vi "process.vi"(8 "error in (no error)":errorcluster, 11 "ConnectionHandler in":refnum<class "ConnectionHandler.lvclass">) -> (0 "error out":errorcluster, 3 "ConnectionHandler":refnum<class "ConnectionHandler.lvclass">)   [LabVIEW 2013, in "MQTT Server.lvlib" / "ConnectionHandler.lvclass"]
uses:
  ConnectionHandler.lvclass
  <vilib>/LabVIEW Open Source Project/MQTT Connection/MQTT_Base/Session/Session.lvclass
  ConnectionHandler.lvclass/ConnectionHandler.ctl
  Session.Server/Session.Server.lvclass
  <vilib>/LabVIEW Open Source Project/MQTT Connection/MQTT_Base/Session/Session.lvclass/Session.ctl
  <vilib>/Utility/error.llb/Clear Errors.vi
  <vilib>/LabVIEW Open Source Project/MQTT Connection/MQTT_Connection/Connection/Connection.lvclass
panel:
  out "Stored Connections":i32
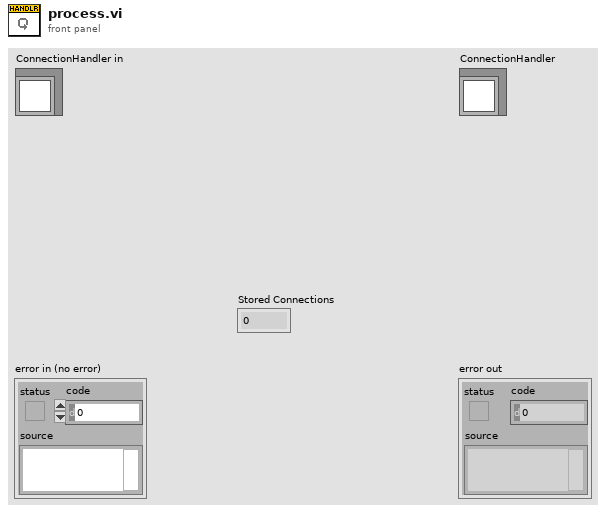
[diagram p1: front panel]
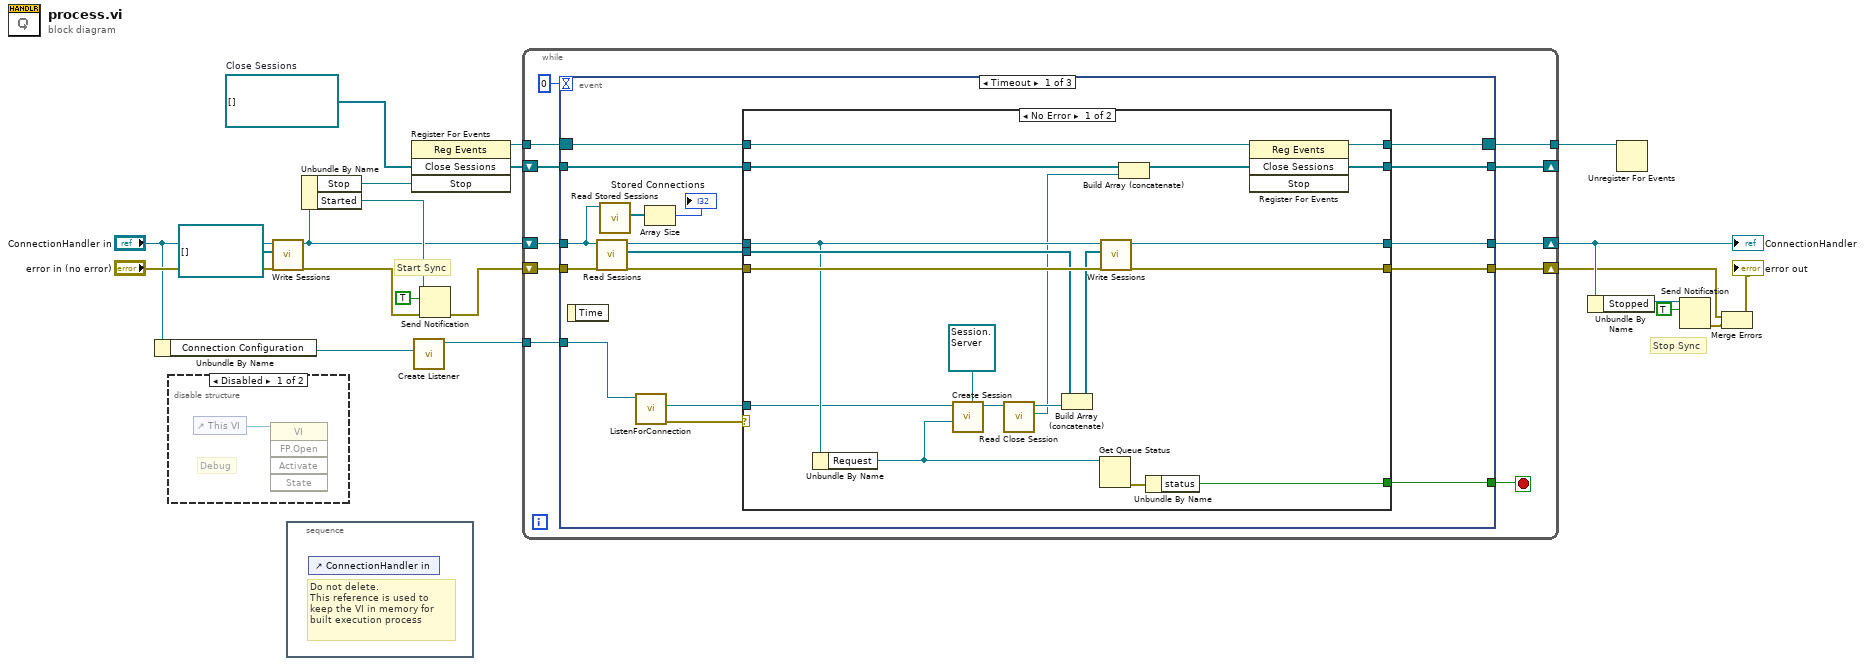
[diagram p0: block diagram]
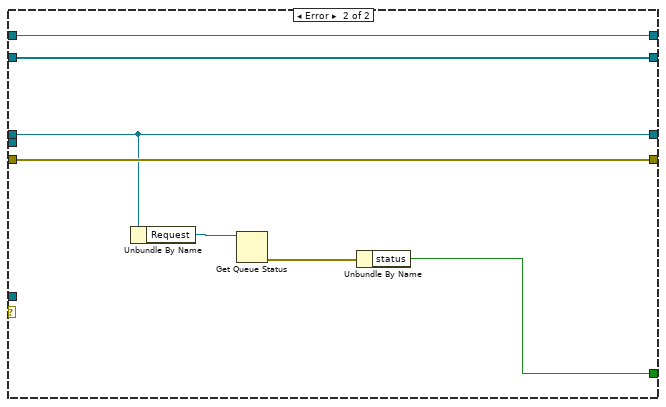
[diagram p3: hidden frame]
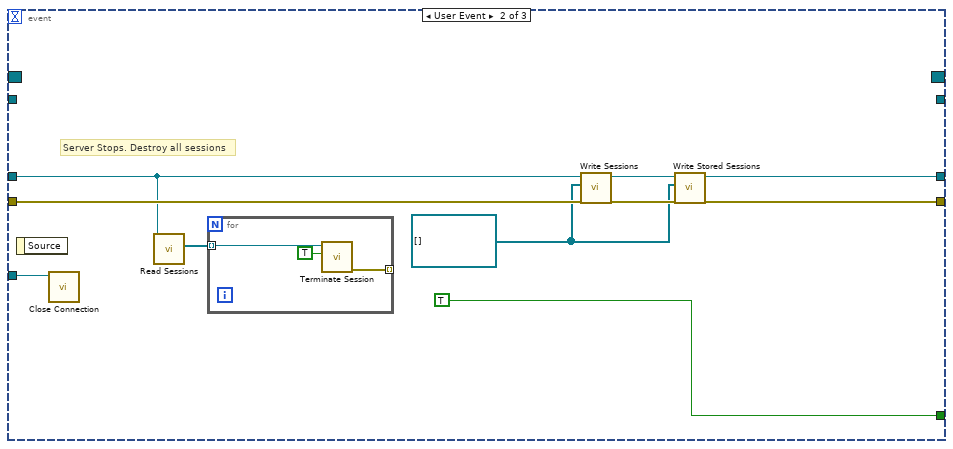
[diagram p4: hidden frame]
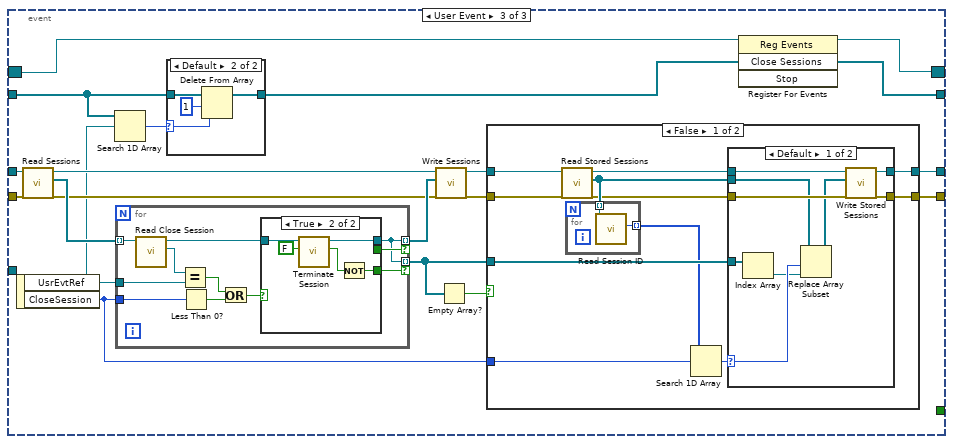
[diagram p5: hidden frame]
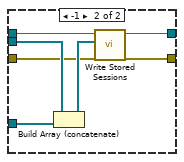
[diagram p7: hidden frame]
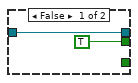
[diagram p9: hidden frame]
diagram:
  w4 = refnum<user-event>[] []  # Close Sessions
  # "Stop Sync"
  # "Start Sync"
  n1 = Unbundle By Name("ConnectionHandler in") -> ("Connection Configuration"=w6:refnum<class "Connection.lvclass">)
  n2 = disable-structure shown="Disabled" {
    frame Disabled {
      # "Debug"
      n3 = control-ref of="This VI"() -> (w20:refnum<vi>)
      n4 = invoke class="VI" method="FP.Open"(reference=w20) -> ()  [unwired: 4 in, 5 out]
    }
    frame Enabled {
    }
  }
  n5 = call "Write Sessions.vi"("Sessions"=refnum<class "Session.lvclass">[] [], "ConnectionHandler in"="ConnectionHandler in") -> ("ConnectionHandler"=w2:refnum<class "ConnectionHandler.lvclass">)  [unwired: 9 in]
  n6 = stacked-sequence {
    frame #0 {
      # "Do not delete.\nThis reference is used to keep the VI in memory for built execution process"
      n7 = control-ref of="ConnectionHandler in"() -> ()  [unwired: 1 out]
    }
  }
  n8 = Unbundle By Name(w2) -> ("Stop"=w19:refnum<user-event>, "Started"=w14:refnum<notifier>)
  n9 = register-events(w4, w19) -> (reference out=w17:refnum<event-registration>)  [unwired: 2 in, 1 out]
  n10 = call <vilib>:"Create Listener.vi"("Connection Configuration"=w6) -> ("Listener"=w5:refnum<class "Connection.lvclass">)  [unwired: 9 in, 1 out]
  n11 = Send Notification(notification=TRUE, notifier=w14, error in (no error)="error in (no error)") -> (error out=w15:errorcluster)  [unwired: 1 out]
  n12 = while {
    shift-right: [w28] -> w13
    shift-left: w2 -> [w27]
    shift-right: [w30] -> w8
    shift-left: w15 -> [w29]
    tunnel: w17 -> [w26]
    tunnel: [w25] -> w18
    tunnel: w5 -> [w23]
    shift-right: [w22] -> _
    shift-left: w4 -> [w21]
    stop <- w24 stop-if-true
    n13 = event shown="[0] Timeout" {
      selector: w26 -> [w35 _ w86]
      dyn-events: [w34 _ w87] -> w25
      timeout: 0 -> [_ _ _]
      tunnel: [w45 w79 w91] -> w30
      tunnel: w29 -> [w47 w79 w90]
      tunnel: [w46 w74 w97] -> w28
      tunnel: w27 -> [w41 w76 w95]
      tunnel: [w44 TRUE _] -> w24
      tunnel: w23 -> [w37 w72 _]
      tunnel: [w33 _ w83] -> w22
      tunnel: w21 -> [w32 _ w85]
      event Timeout {
        n14 = event-data() -> ()  [unwired: 1 in, 1 out]
        n15 = call "Read Sessions.vi"("ConnectionHandler in"=w41) -> ("Sessions"=w42:refnum<class "Session.lvclass">[], "ConnectionHandler"=w43:refnum<class "ConnectionHandler.lvclass">)  [unwired: 9 in]
        n16 = call "Read Stored Sessions.vi"("ConnectionHandler in"=w41) -> ("Stored Sessions"=w40:refnum<class "Session.lvclass">[])  [unwired: 9 in, 1 out]
        n17 = call <vilib>:"ListenForConnection.vi"("Listener"=w37) -> ("error out"=w38:errorcluster, "Connection"=w39:refnum<class "Connection.lvclass">)  [unwired: 7 in, 2 out]
        n18 = Array Size(array=w40) -> (size(s)=→"Stored Connections":i32)
        n19 = case shown="No Error" w38 {
          tunnel: w43 -> [w59 w70]
          tunnel: w47 -> [w64 w71]
          tunnel: [w63 w70] -> w46
          tunnel: [w64 w71] -> w45
          tunnel: [w61 w67] -> w44
          tunnel: w42 -> [w60 _]
          tunnel: w39 -> [w57 _]
          tunnel: w35 -> [w55 w66]
          tunnel: [w54 w66] -> w34
          tunnel: [w48 w65] -> w33
          tunnel: w32 -> [w49 w65]
          frame No Error {
            n20 = Unbundle By Name(w59) -> ("Request"=w56:refnum<queue>)
            n21 = call <vilib>:"Create Session.vi"("Session in"=refnum<class "Session.Server.lvclass"> refnum ("MQTT Server.lvlib:Session.Server.lvclass"), "Request"=w56, "Connection"=w57) -> ("Session"=w52:refnum<class "Session.Server.lvclass">)  [unwired: 7 in, 1 out]
            n22 = call <vilib>:"Read Close Session.vi"("Session in"=w52) -> ("Close Session"=w50:refnum<user-event>, "Session out"=w51:refnum<class "Session.Server.lvclass">)  [unwired: 8 in, 1 out]
            n23 = Build Array (concatenate)(w60, w51) -> (w53:refnum<class "Session.lvclass">[])
            n24 = Get Queue Status(queue=w56) -> (error out=w62:errorcluster)  [unwired: 2 in, 7 out]
            n25 = call "Write Sessions.vi"("Sessions"=w53, "ConnectionHandler in"=w59) -> ("ConnectionHandler"=w63:refnum<class "ConnectionHandler.lvclass">)  [unwired: 9 in]
            n26 = Build Array (concatenate)(w49, w50) -> (w48:refnum<user-event>[])
            n27 = Unbundle By Name(w62) -> ("status"=w61:bool)
            n28 = register-events(reference=w55, w48) -> (reference out=w54:refnum<event-registration>)  [unwired: 2 in, 1 out]
          }
          frame Error {
            n29 = Unbundle By Name(w70) -> ("Request"=w69:refnum<queue>)
            n30 = Get Queue Status(queue=w69) -> (error out=w68:errorcluster)  [unwired: 2 in, 7 out]
            n31 = Unbundle By Name(w68) -> ("status"=w67:bool)
          }
        }
      }
      event User Event {
        w73 = refnum<class "Session.lvclass">[] [] ("Sessions")
        # "Server Stops. Destroy all sessions"
        n32 = event-data() -> ()  [unwired: 1 in, 1 out]
        n33 = call <vilib>:"Close Connection.vi"("Connection in"=w72) -> ()  [unwired: 9 in, 2 out]
        n34 = call "Read Sessions.vi"("ConnectionHandler in"=w76) -> ("Sessions"=w77:refnum<class "Session.lvclass">[])  [unwired: 9 in, 1 out]
        n35 = for {
          tunnel: w77 -> [w82] mode=indexing
          tunnel: [w81] -> _ mode=indexing
          n36 = call <vilib>:"Terminate Session.vi"("Destroy (T)"=TRUE, "Session in"=w82) -> ("error out"=w81:errorcluster)  [unwired: 7 in, 2 out]
        }
        n37 = call "Write Sessions.vi"("Sessions"=w73, "ConnectionHandler in"=w76) -> ("ConnectionHandler"=w75:refnum<class "ConnectionHandler.lvclass">)  [unwired: 9 in]
        n38 = call "Write Stored Sessions.vi"("Stored Sessions"=w73, "ConnectionHandler in"=w75) -> ("ConnectionHandler"=w74:refnum<class "ConnectionHandler.lvclass">)  [unwired: 9 in]
      }
      event User Event {
        n39 = event-data() -> ("UsrEvtRef"=w88:refnum<user-event>, "CloseSession"=w89:i32)  [unwired: 1 in]
        n40 = call "Read Sessions.vi"("ConnectionHandler in"=w95) -> ("Sessions"=w99:refnum<class "Session.lvclass">[], "ConnectionHandler"=w94:refnum<class "ConnectionHandler.lvclass">)  [unwired: 9 in]
        n41 = Search 1D Array(1D array=w85, element=w88) -> (index of element=w84:i32)  [unwired: 1 in]
        n42 = for {
          tunnel: w99 -> [w133] mode=indexing
          tunnel: [w139] -> w98 mode=indexing if=w143
          tunnel: w89 -> [w141]
          tunnel: [w139] -> w93 mode=indexing if=w138
          tunnel: w88 -> [w136]
          n43 = call <vilib>:"Read Close Session.vi"("Session in"=w133) -> ("Close Session"=w134:refnum<user-event>, "Session out"=w137:refnum<class "Session.lvclass">)  [unwired: 8 in, 1 out]
          n44 = Equal?(x=w134, y=w136) -> (x = y?=w135:bool)
          n45 = Less Than 0?(x=w141) -> (x < 0?=w142:bool)
          n46 = Or(x=w135, y=w142) -> (x .or. y?=w140:bool)
          n47 = case shown="True" w140 {
            tunnel: w137 -> [w145 w150]
            tunnel: [w145 w149] -> w139
            tunnel: [TRUE _] -> w143
            tunnel: [_ w146] -> w138
            frame False {
            }
            frame True {
              n48 = call <vilib>:"Terminate Session.vi"("Destroy (T)"=FALSE, "Session in"=w150) -> ("Destroyed"=w147:bool, "Session out"=w149:refnum<class "Session.lvclass">)  [unwired: 7 in, 1 out]
              n49 = Not(x=w147) -> (.not. x?=w146:bool)
            }
          }
        }
        n50 = case shown="Default" w84 {
          selector: w84 -> [_ w101]
          tunnel: w85 -> [w100 w104]
          tunnel: [w100 w102] -> w83
          frame -1 {
          }
          frame Default {
            n51 = Delete From Array(array=w104, length=1, index=w101) -> (array with subset deleted=w102:refnum<user-event>[])  [unwired: 1 out]
          }
        }
        n52 = call "Write Sessions.vi"("Sessions"=w98, "ConnectionHandler in"=w94) -> ("ConnectionHandler"=w96:refnum<class "ConnectionHandler.lvclass">)  [unwired: 9 in]
        n53 = Empty Array?(array=w93) -> (empty?=w92:bool)
        n54 = case shown="False" w92 {
          tunnel: [w114 w132] -> w97
          tunnel: w96 -> [w113 w132]
          tunnel: w93 -> [w111 _]
          tunnel: [w105 w131] -> w91
          tunnel: w90 -> [w106 w131]
          tunnel: w89 -> [w108 _]
          frame False {
            n55 = call "Read Stored Sessions.vi"("ConnectionHandler in"=w113) -> ("Stored Sessions"=w110:refnum<class "Session.lvclass">[], "ConnectionHandler"=w112:refnum<class "ConnectionHandler.lvclass">)  [unwired: 9 in]
            n56 = for {
              tunnel: w110 -> [w130] mode=indexing
              tunnel: [w129] -> w109 mode=indexing
              n57 = call <vilib>:"Read Session ID.vi"("Session in"=w130) -> ("Session ID"=w129:i32)  [unwired: 8 in, 2 out]
            }
            n58 = Search 1D Array(1D array=w109, element=w108) -> (index of element=w107:i32)  [unwired: 1 in]
            n59 = case shown="Default" w107 {
              selector: w107 -> [w118 _]
              tunnel: [w122 w128] -> w114
              tunnel: w112 -> [w120 w127]
              tunnel: w111 -> [w117 w125]
              tunnel: w110 -> [w119 w124]
              tunnel: w106 -> [w121 w123]
              tunnel: [w121 w123] -> w105
              frame Default {
                n60 = Index Array(array=w117) -> (element=w116:refnum<class "Session.lvclass">)  [unwired: 1 in]
                n61 = Replace Array Subset(array=w119, new element=w116, index=w118) -> (w115:refnum<class "Session.lvclass">[])
                n62 = call "Write Stored Sessions.vi"("Stored Sessions"=w115, "ConnectionHandler in"=w120) -> ("ConnectionHandler"=w122:refnum<class "ConnectionHandler.lvclass">)  [unwired: 9 in]
              }
              frame -1 {
                n63 = Build Array (concatenate)(w124, w125) -> (w126:refnum<class "Session.lvclass">[])
                n64 = call "Write Stored Sessions.vi"("Stored Sessions"=w126, "ConnectionHandler in"=w127) -> ("ConnectionHandler"=w128:refnum<class "ConnectionHandler.lvclass">)  [unwired: 9 in]
              }
            }
          }
          frame True {
          }
        }
        n65 = register-events(reference=w86, w83) -> (reference out=w87:refnum<event-registration>)  [unwired: 2 in, 1 out]
      }
    }
  }
  "ConnectionHandler" <- w13
  n66 = Unbundle By Name(w13) -> ("Stopped"=w12:refnum<notifier>)
  n67 = Unregister For Events(event registration refnum=w18) -> ()  [unwired: 1 in, 1 out]
  n68 = Send Notification(notification=TRUE, notifier=w12) -> (error out=w9:errorcluster)  [unwired: 1 in, 1 out]
  n69 = Merge Errors(w8, w9) -> (→"error out":errorcluster)
